vi "Destroy.vi"(8 "error in (no error)":errorcluster, 11 "SMO":refnum<class "SMO.lvclass">) -> (0 "error out":errorcluster)   [LabVIEW 2013, in "SMO.lvclass"]
doc: "Destructor\n\nNote 01: This method is overridable by descendant\nNote 02: When overridden, Call Parent Method is required\n\n---------------------------------------------------------------\nJKI State Machine Objects™\nhttp://jki.net/state-machine-objects/\nCopyright (C) 2005-2015, JKI <info@jki.net>\nALL RIGHTS RESERVED"
uses:
  SMO.lvclass
  Registry/Registry-SMO.lvclass
panel:
  # "For instructions on how to use the JKI State Machine Objects, examples and video tutorials, visit:\nhttp://jki.net/state-machine-objects/\n\nJKI State Machine Objects™\nhttp://jki.net/state-machine-objects/\nCopyright (C) 2005-2015, JKI <info@jki.net>\nALL RIGHTS RESERVED"
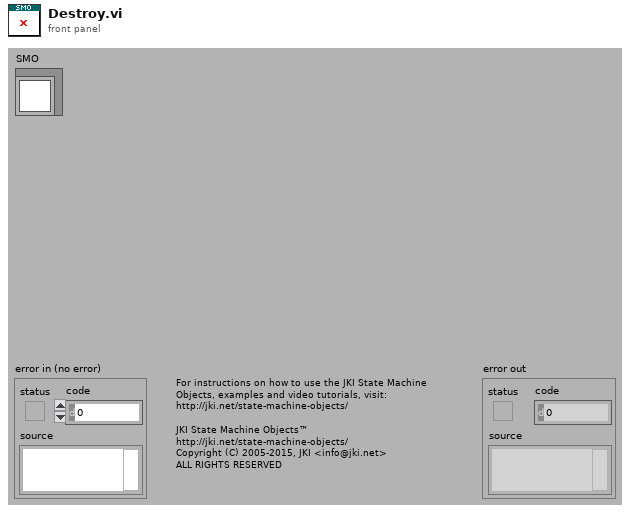
[diagram p1: front panel]
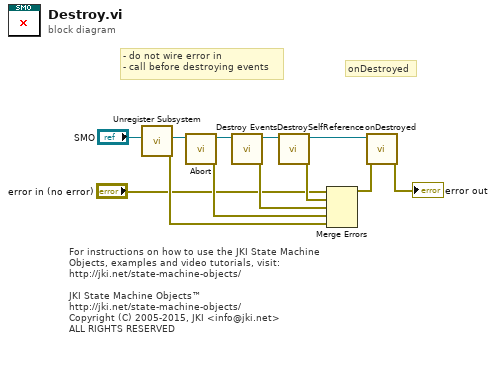
[diagram p0: block diagram]
diagram:
  # "onDestroyed"
  # "- do not wire error in\n- call before destroying events"
  # "For instructions on how to use the JKI State Machine Objects, examples and video tutorials, visit:\nhttp://jki.net/state-machine-objects/\n\nJKI State Machine Objects™\nhttp://jki.net/state-machine-objects/\nCopyright (C) 2005-2015, JKI <info@jki.net>\nALL RIGHTS RESERVED"
  n1 = call "Unregister Subsystem.vi"("JKI SMO"="SMO") -> ("error out"=w7:errorcluster, "JKI SMO out"=w11:refnum<class "SMO.lvclass">)  [unwired: 9 in]
  n2 = call "Abort.vi"("SMO"=w11) -> ("error out"=w8:errorcluster, "SMO out"=w10:refnum<class "SMO.lvclass">)  [unwired: 9 in]
  n3 = call "Destroy Events.vi"("SMO"=w10) -> ("error out"=w9:errorcluster, "SMO out"=w6:refnum<class "SMO.lvclass">)  [unwired: 9 in]
  n4 = call-dynamic "DestroySelfReference.vi"("SMO"=w6) -> ("error out"=w5:errorcluster, "SMO out"=w3:refnum<class "SMO.lvclass">)  [unwired: 9 in]
  n5 = Merge Errors("error in (no error)", w5, w9, w8, w7) -> (w2:errorcluster)
  n6 = call-dynamic "onDestroyed.vi"("error in (no error)"=w2, "SMO"=w3) -> ("error out"=→"error out":errorcluster)  [unwired: 9 in]
